vi "Set Index.vi"(8 "error in (no error)":errorcluster, 10 "Index (-1)":i32=-1, 11 "CO2 Actor in":refnum<class "CO2 Actor.lvclass">) -> (0 "error out":errorcluster, 3 "CO2 Actor out":refnum<class "CO2 Actor.lvclass">)   [LabVIEW 2015, in "cRIO-Carbondioxide.lvlib" / "CO2-Actor.lvlib" / "CO2 Actor.lvclass"]
uses:
  CO2 Actor.lvclass
  CO2 Actor.lvclass/CO2 Actor.ctl
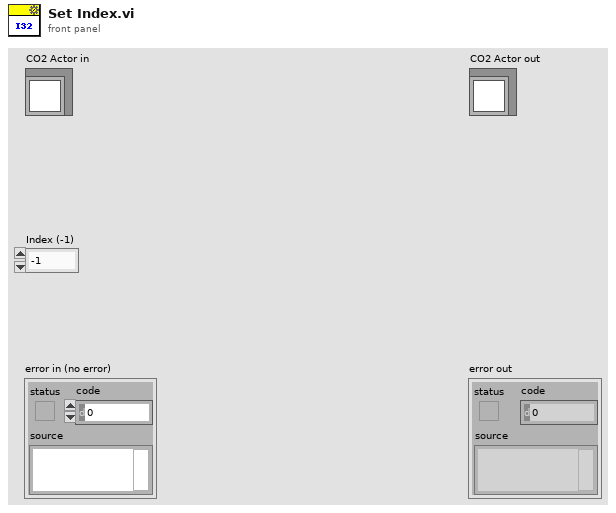
[diagram p1: front panel]
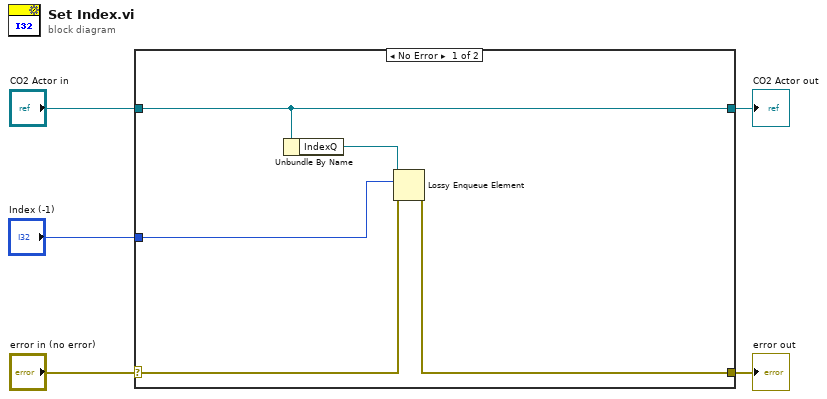
[diagram p0: block diagram]
diagram:
  n1 = case shown="No Error" "error in (no error)" {
    selector: "error in (no error)" -> [w9 w12]
    tunnel: [w7 w12] -> w4
    tunnel: [w6 w11] -> w2
    tunnel: "CO2 Actor in" -> [w6 w11]
    tunnel: "Index (-1)" -> [w8 _]
    frame No Error {
      n2 = Unbundle By Name(w6) -> ("IndexQ"=w10:refnum<queue>)
      n3 = Lossy Enqueue Element(queue=w10, element=w8, error in (no error)=w9) -> (error out=w7:errorcluster)  [unwired: 3 out]
    }
    frame Error {
    }
  }
  "error out" <- w4
  "CO2 Actor out" <- w2
